vi "Set Measurement.vi"(6 "Escala":dbl, 8 "error in (no error)":errorcluster, 9 "Range ON/OFF":bool, 10 "Grandeza Elétrica":string, 11 "34410A in":refnum<class "34410A.lvclass">) -> (0 "error out":errorcluster, 3 "34410A out":refnum<class "34410A.lvclass">)   [LabVIEW 2015, in "34410A.lvclass"]
uses:
  34410A.lvclass
  <instrlib>/Agilent 34401/Agilent 34401.lvlib
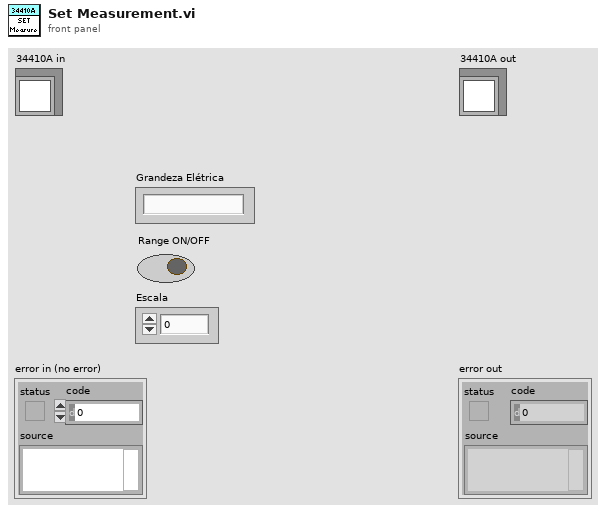
[diagram p1: front panel]
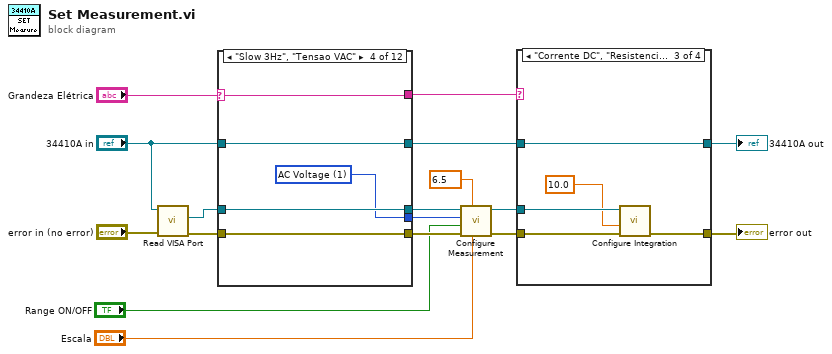
[diagram p0: block diagram]
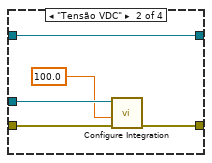
[diagram p3: hidden frame]
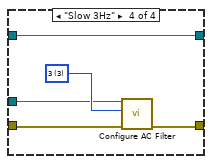
[diagram p4: hidden frame]
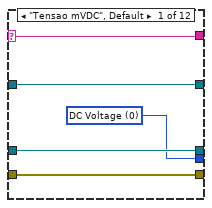
[diagram p5: hidden frame]
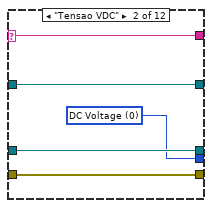
[diagram p6: hidden frame]
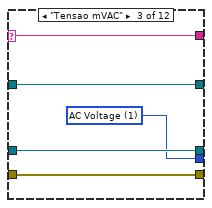
[diagram p7: hidden frame]
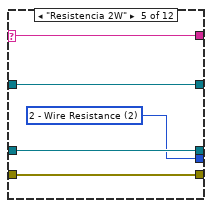
[diagram p8: hidden frame]
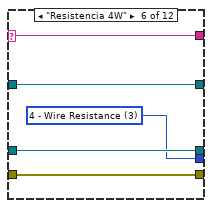
[diagram p9: hidden frame]
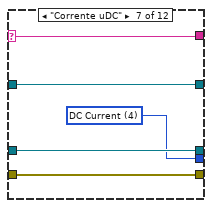
[diagram p10: hidden frame]
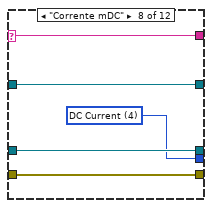
[diagram p11: hidden frame]
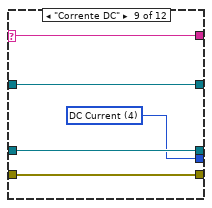
[diagram p12: hidden frame]
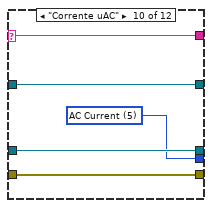
[diagram p13: hidden frame]
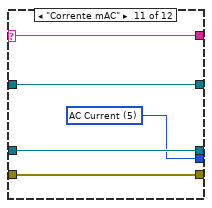
[diagram p14: hidden frame]
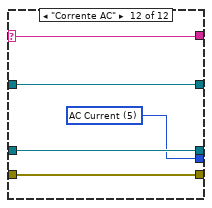
[diagram p15: hidden frame]
diagram:
  w10 = 6.5 items=["4.5"=4.5, "5.5"=5.5, "6.5"=6.5] ("Manual Resolution (5.5 Digits)")
  n1 = call-dynamic "Read VISA Port.vi"("error in (no error)"="error in (no error)", "Device in"="34410A in") -> ("error out"=w16:errorcluster, "VISA Port"=w15:refnum<visa-resource-name>)  [unwired: 7 in, 1 out]
  n2 = case shown="\"Slow 3Hz\", \"Tensao VAC\"" "Grandeza Elétrica" {
    selector: "Grandeza Elétrica" -> [w18 w23 w28 w33 w38 w43 w48 w53 w58 w63 w68 w73]
    tunnel: w16 -> [w21 w26 w31 w36 w41 w46 w51 w56 w61 w66 w71 w76]
    tunnel: w15 -> [w22 w27 w32 w37 w42 w47 w52 w57 w62 w67 w72 w77]
    tunnel: [w22 w27 w32 w37 w42 w47 w52 w57 w62 w67 w72 w77] -> w14
    tunnel: [w21 w26 w31 w36 w41 w46 w51 w56 w61 w66 w71 w76] -> w13
    tunnel: "34410A in" -> [w20 w25 w30 w35 w40 w45 w50 w55 w60 w65 w70 w75]
    tunnel: [w20 w25 w30 w35 w40 w45 w50 w55 w60 w65 w70 w75] -> w6
    tunnel: [w19 w24 w29 w34 w39 w44 w49 w54 w59 w64 w69 w74] -> w11
    tunnel: [w18 w23 w28 w33 w38 w43 w48 w53 w58 w63 w68 w73] -> w7
    frame "Tensao mVDC", Default {
      w19 = u16 0 items=["DC Voltage", "AC Voltage", "2 - Wire Resistance", "4 - Wire Resistance", "DC Current", "AC Current", "Frequency", "Period", "Continuity", "Diode Checking", "VDC:VDC Ratio", "Temperature", "Capacitance"] ("Function (0: DC Voltage)")
    }
    frame "Tensao VDC" {
      w24 = u16 0 items=["DC Voltage", "AC Voltage", "2 - Wire Resistance", "4 - Wire Resistance", "DC Current", "AC Current", "Frequency", "Period", "Continuity", "Diode Checking", "VDC:VDC Ratio", "Temperature", "Capacitance"] ("Function (0: DC Voltage)")
    }
    frame "Tensao mVAC" {
      w29 = u16 1 items=["DC Voltage", "AC Voltage", "2 - Wire Resistance", "4 - Wire Resistance", "DC Current", "AC Current", "Frequency", "Period", "Continuity", "Diode Checking", "VDC:VDC Ratio", "Temperature", "Capacitance"] ("Function (0: DC Voltage)")
    }
    frame "Slow 3Hz", "Tensao VAC" {
      w34 = u16 1 items=["DC Voltage", "AC Voltage", "2 - Wire Resistance", "4 - Wire Resistance", "DC Current", "AC Current", "Frequency", "Period", "Continuity", "Diode Checking", "VDC:VDC Ratio", "Temperature", "Capacitance"] ("Function (0: DC Voltage)")
    }
    frame "Resistencia 2W" {
      w39 = u16 2 items=["DC Voltage", "AC Voltage", "2 - Wire Resistance", "4 - Wire Resistance", "DC Current", "AC Current", "Frequency", "Period", "Continuity", "Diode Checking", "VDC:VDC Ratio", "Temperature", "Capacitance"] ("Function (0: DC Voltage)")
    }
    frame "Resistencia 4W" {
      w44 = u16 3 items=["DC Voltage", "AC Voltage", "2 - Wire Resistance", "4 - Wire Resistance", "DC Current", "AC Current", "Frequency", "Period", "Continuity", "Diode Checking", "VDC:VDC Ratio", "Temperature", "Capacitance"] ("Function (0: DC Voltage)")
    }
    frame "Corrente uDC" {
      w49 = u16 4 items=["DC Voltage", "AC Voltage", "2 - Wire Resistance", "4 - Wire Resistance", "DC Current", "AC Current", "Frequency", "Period", "Continuity", "Diode Checking", "VDC:VDC Ratio", "Temperature", "Capacitance"] ("Function (0: DC Voltage)")
    }
    frame "Corrente mDC" {
      w54 = u16 4 items=["DC Voltage", "AC Voltage", "2 - Wire Resistance", "4 - Wire Resistance", "DC Current", "AC Current", "Frequency", "Period", "Continuity", "Diode Checking", "VDC:VDC Ratio", "Temperature", "Capacitance"] ("Function (0: DC Voltage)")
    }
    frame "Corrente DC" {
      w59 = u16 4 items=["DC Voltage", "AC Voltage", "2 - Wire Resistance", "4 - Wire Resistance", "DC Current", "AC Current", "Frequency", "Period", "Continuity", "Diode Checking", "VDC:VDC Ratio", "Temperature", "Capacitance"] ("Function (0: DC Voltage)")
    }
    frame "Corrente uAC" {
      w64 = u16 5 items=["DC Voltage", "AC Voltage", "2 - Wire Resistance", "4 - Wire Resistance", "DC Current", "AC Current", "Frequency", "Period", "Continuity", "Diode Checking", "VDC:VDC Ratio", "Temperature", "Capacitance"] ("Function (0: DC Voltage)")
    }
    frame "Corrente mAC" {
      w69 = u16 5 items=["DC Voltage", "AC Voltage", "2 - Wire Resistance", "4 - Wire Resistance", "DC Current", "AC Current", "Frequency", "Period", "Continuity", "Diode Checking", "VDC:VDC Ratio", "Temperature", "Capacitance"] ("Function (0: DC Voltage)")
    }
    frame "Corrente AC" {
      w74 = u16 5 items=["DC Voltage", "AC Voltage", "2 - Wire Resistance", "4 - Wire Resistance", "DC Current", "AC Current", "Frequency", "Period", "Continuity", "Diode Checking", "VDC:VDC Ratio", "Temperature", "Capacitance"] ("Function (0: DC Voltage)")
    }
  }
  n3 = call <instrlib>:"Configure Measurement.vi"("Manual Range (1.00)"="Escala", "Manual Resolution (5.5 Digits)"=w10, "error in (no error)"=w13, "Enable Auto Range (T: Enable)"="Range ON/OFF", "Function (0: DC Voltage)"=w11, "VISA resource name"=w14) -> ("error out"=w4:errorcluster, "VISA resource name out"=w5:refnum<visa-resource-name>)  [unwired: 4 in]
  n4 = case shown="\"Corrente DC\", \"Resistencia 2W\", \"Resistencia 4W\"" w7 {
    tunnel: w6 -> [w79 w84 w89 w94]
    tunnel: [w79 w84 w89 w94] -> w8
    tunnel: w5 -> [_ w83 w88 w92]
    tunnel: w4 -> [w78 w81 w86 w91]
    tunnel: [w78 w80 w85 w90] -> w3
    frame "Tensão mVDC", Default {
    }
    frame "Tensão VDC" {
      w82 = 100.0 items=["0.001"=0.001, "0.002"=0.002, "0.006"=0.006, "0.02"=0.02, "0.06"=0.06, "0.2"=0.2, "1"=1.0, "10"=10.0, "100"=100.0] ("Integration Time (1 PLCs)")
      n5 = call <instrlib>:"Configure Integration.vi"("error in (no error)"=w81, "Integration Time (1 PLCs)"=w82, "VISA resource name"=w83) -> ("error out"=w80:errorcluster)  [unwired: 7 in, 1 out]
    }
    frame "Corrente DC", "Resistencia 2W", "Resistencia 4W" {
      w87 = 10.0 items=["0.001"=0.001, "0.002"=0.002, "0.006"=0.006, "0.02"=0.02, "0.06"=0.06, "0.2"=0.2, "1"=1.0, "10"=10.0, "100"=100.0] ("Integration Time (1 PLCs)")
      n6 = call <instrlib>:"Configure Integration.vi"("error in (no error)"=w86, "Integration Time (1 PLCs)"=w87, "VISA resource name"=w88) -> ("error out"=w85:errorcluster)  [unwired: 7 in, 1 out]
    }
    frame "Slow 3Hz" {
      w93 = 3 items=["3"=3, "20"=20, "200"=200] ("AC Filter Bandwidth (20 Hz)")
      n7 = call <instrlib>:"Configure AC Filter.vi"("error in (no error)"=w91, "AC Filter Bandwidth (20 Hz)"=w93, "VISA resource name"=w92) -> ("error out"=w90:errorcluster)  [unwired: 7 in, 1 out]
    }
  }
  "error out" <- w3
  "34410A out" <- w8
